vi "receiver_tcp.vi"(1 "stop":bool, 2 "String":string) -> (0 "Cluster":cluster{dbl[], dbl[], dbl[], dbl[]})   [LabVIEW 2013]
panel:
  in  "Server Closed":string="The server VI closed the connection."
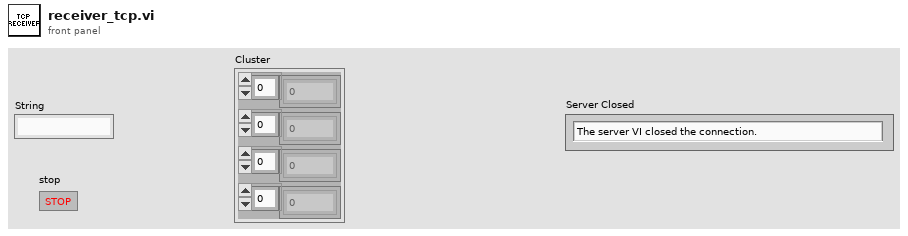
[diagram p1: front panel]
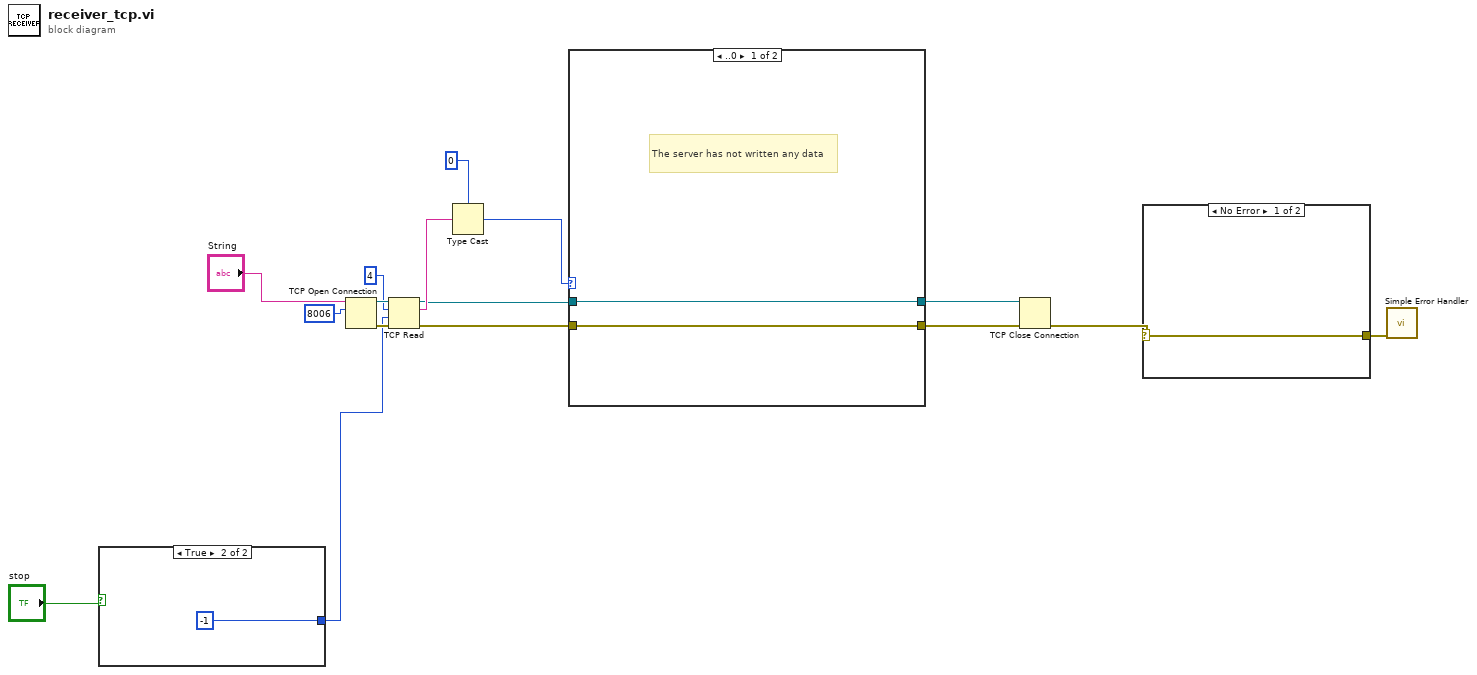
[diagram p0: block diagram]
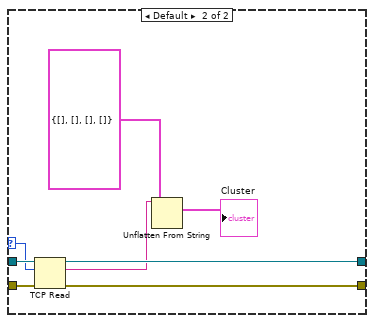
[diagram p2: hidden frame]
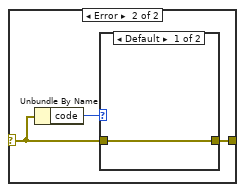
[diagram p3: hidden frame]
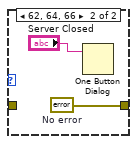
[diagram p4: hidden frame]
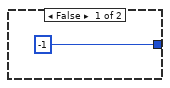
[diagram p5: hidden frame]
diagram:
  n1 = case shown="True" "stop" {
    tunnel: [-1 -1] -> w8
    frame False {
    }
    frame True {
    }
  }
  n2 = TCP Open Connection(address="String", remote port or service name=8006) -> (connection ID=w14:refnum<k5>, error out=w15:errorcluster)  [unwired: 3 in]
  n3 = TCP Read(connection ID=w14, bytes to read=4, error in (no error)=w15, 9:w8) -> (connection ID out=w4:refnum<k5>, data out=w11:string, error out=w2:errorcluster)  [unwired: 1 in]
  n4 = Type Cast(type=0, x=w11) -> (*(type *) &x=w5:i32)
  n5 = case shown="..0" w5 {
    selector: w5 -> [_ w24]
    tunnel: w4 -> [w20 w28]
    tunnel: w2 -> [w19 w27]
    tunnel: [w20 w26] -> w3
    tunnel: [w19 w25] -> w1
    frame ..0 {
      # "The server has not written any data"
    }
    frame Default {
      n6 = TCP Read(connection ID=w28, bytes to read=w24, error in (no error)=w27) -> (connection ID out=w26:refnum<k5>, data out=w21:string, error out=w25:errorcluster)  [unwired: 2 in]
      n7 = Unflatten From String(type=cluster{dbl[], dbl[], dbl[], dbl[]} {[], [], [], []}, binary string=w21) -> (value=→"Cluster":cluster{dbl[], dbl[], dbl[], dbl[]})  [unwired: 3 in, 2 out]
    }
  }
  n8 = TCP Close Connection(connection ID=w3, error in (no error)=w1) -> (error out=w6:errorcluster)  [unwired: 1 in, 1 out]
  n9 = case shown="No Error" w6 {
    selector: w6 -> [w29 w31]
    tunnel: [w29 w30] -> w7
    frame No Error {
    }
    frame Error {
      n10 = Unbundle By Name(w31) -> ("code"=w32:i32)
      n11 = case shown="Default" w32 {
        tunnel: w31 -> [w33 _]
        tunnel: [w33 w35] -> w30
        frame Default {
        }
        frame 62, 64, 66 {
          w35 = errorcluster {"status"=FALSE, "code"=0, "source"=""}  # No error
          n12 = One Button Dialog(message="Server Closed") -> ()  [unwired: 1 in, 1 out]
        }
      }
    }
  }
  n13 = call <vilib>:"Simple Error Handler.vi"("error in (no error)"=w7) -> ()  [unwired: 4 in, 5 out]
